vi "SyncData.vi"(8 "ErrorIn":errorcluster, 10 "CmdData":variant, 11 "YActorIn":refnum<class>) -> (0 "ErrorOut":errorcluster, 2 "ReplyData":variant, 3 "YActorOut":refnum<class>, 4 "Exit":bool)   [LabVIEW 2021, in "YActor.lvclass"]
uses:
  YActor.lvclass
  YActor.lvclass/YActor.ctl
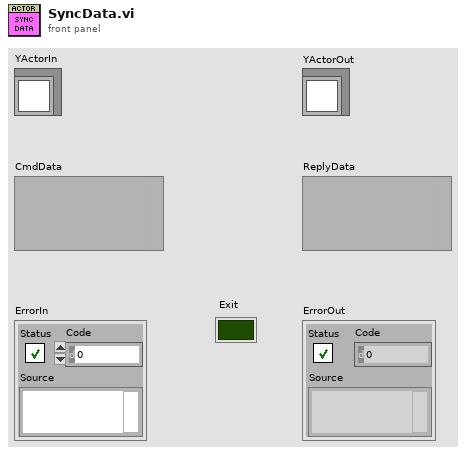
[diagram p1: front panel]
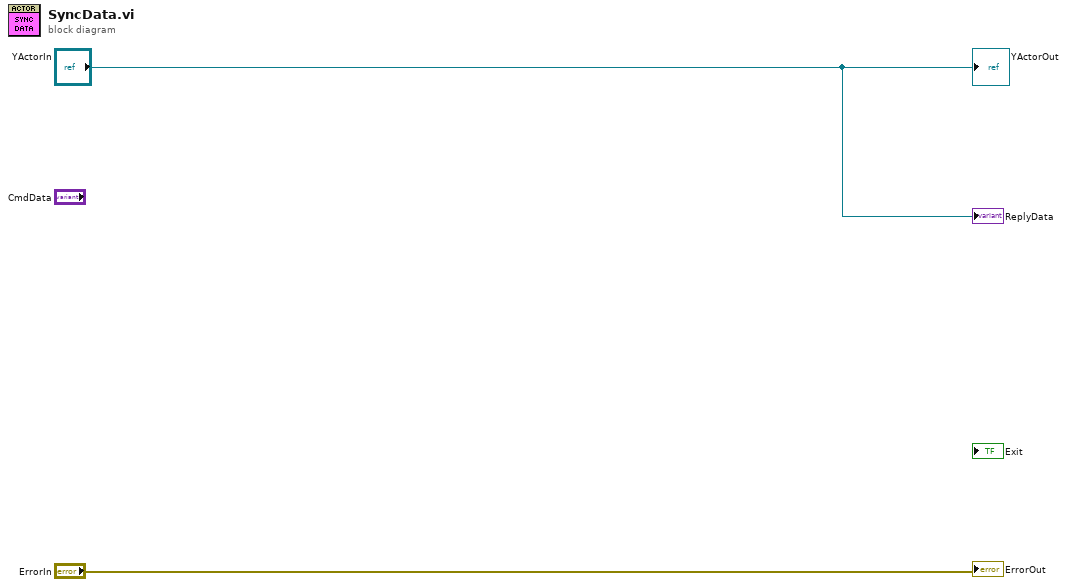
[diagram p0: block diagram]
diagram:
  "ErrorOut" <- "ErrorIn"
  "YActorOut" <- "YActorIn"
  "ReplyData" <- "YActorIn"
